vi "Zernike_to_Motion.vi"(0 "HasoSlopes in":refnum<class "HasoSlopes.lvclass">, 1 "CorrectionDataManager (const)":refnum<class "CorrectionDataManager.lvclass">, 2 "Pupil (const)":refnum<class "Pupil.lvclass">, 3 "WavefrontCorrector in":refnum<class "WavefrontCorrector.lvclass">, 4 "ComputePhaseSet":refnum<class "ComputePhaseSet.lvclass">, 5 "error in (no error)":errorcluster, 6 "radius":sgl, 7 "ModalCoef (const)":refnum<class "ModalCoef.lvclass">, 8 "center":T1, 9 "Prefs in":T2={"Number of kept modes"=32, "Tilt filtering"=FALSE}, 10 "ZernikeArray":dbl[](array[numeric])) -> (12 "CorrectionDataManager out":refnum<class "CorrectionDataManager.lvclass">, 13 "Delta commands 2":sgl[](graph), 14 "HasoSlopes out":refnum<class "HasoSlopes.lvclass">, 15 "Pupil (dup)":refnum<class "Pupil.lvclass">, 16 "WavefrontCorrector out":refnum<class "WavefrontCorrector.lvclass">, 17 "ComputePhaseSet (dup)":refnum<class "ComputePhaseSet.lvclass">, 18 "ModalCoef.lvclass (dup)":refnum<class "ModalCoef.lvclass">, 19 "error out":errorcluster)   [LabVIEW 2020, in "ILAO_BeamShaper.lvclass"]
uses:
  ILAO_BeamShaper.lvclass
  HASO4_3/WaveKit/Controls/InteractionMatrixToCommandMatrixParameters.ctl
  HASO4_3/WaveKit/Classes/Pupil/Pupil.lvclass
  HASO4_3/WaveKit/Classes/WavefrontCorrector/WavefrontCorrector.lvclass
  HASO4_3/WaveKit/Classes/ModalCoef/ModalCoef.lvclass
  HASO4_3/WaveKit/Classes/ComputePhaseSet/ComputePhaseSet.lvclass
  HASO4_3/WaveKit/Classes/CorrectionDataManager/CorrectionDataManager.lvclass
  HASO4_3/WaveKit/Classes/HasoSlopes/HasoSlopes.lvclass
  HASO4_3/WaveKit/Controls/Point2Df.ctl
  HASO4_3/WaveKit/Controls/ZernikeModalPrefs.ctl
  HASO4_3/WaveKit/Controls/ZernikeProjectionPupilSetup.ctl
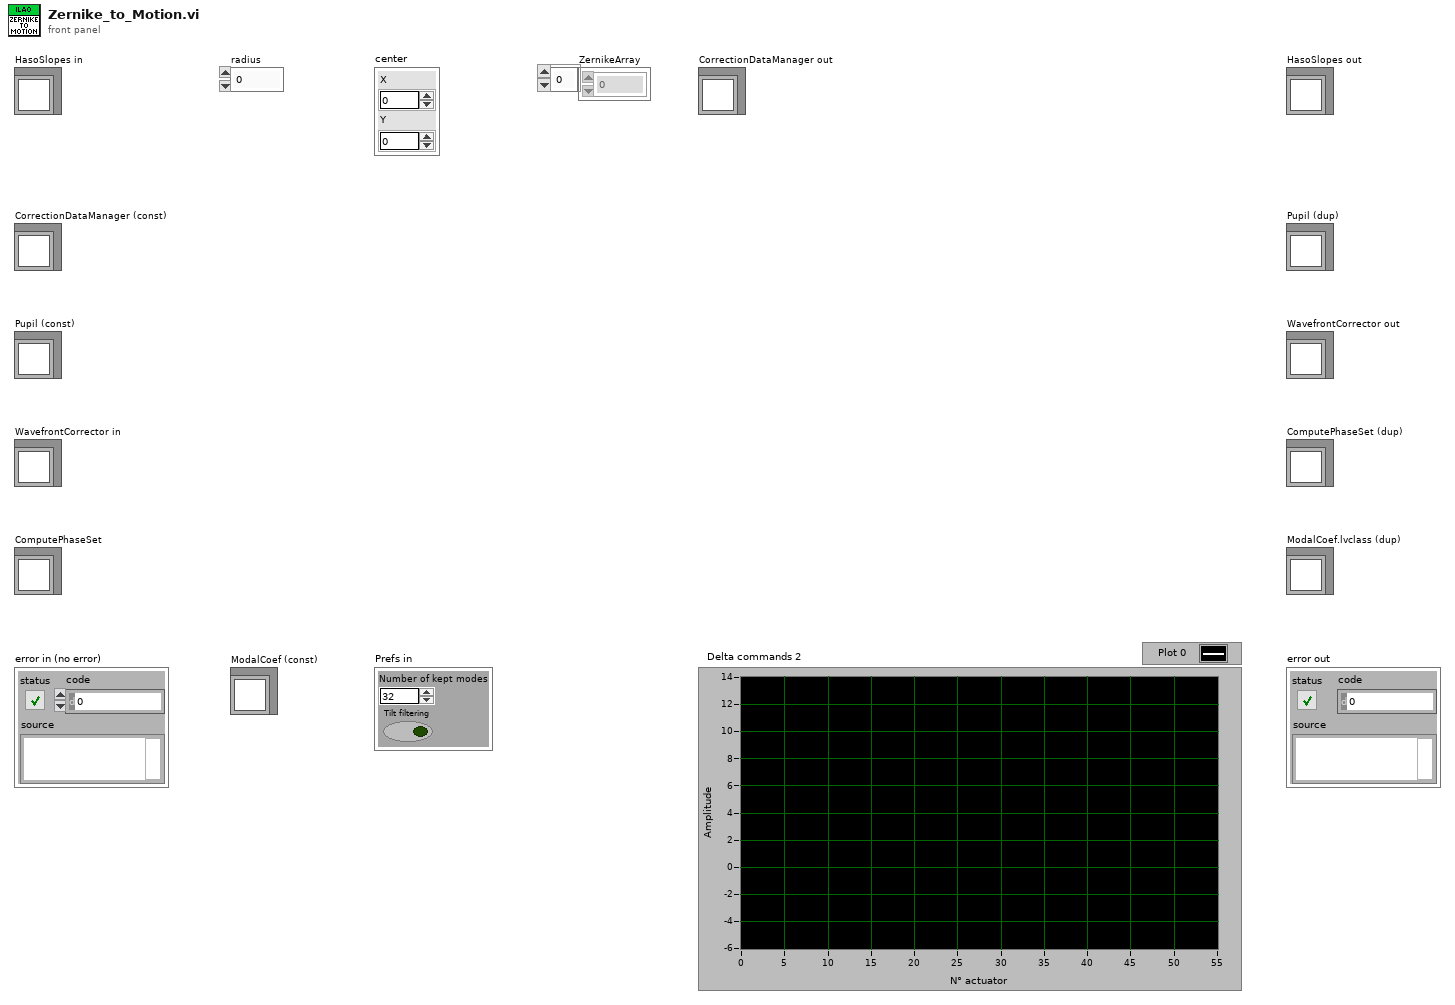
[diagram p1: front panel]
types:
  T1 = typedef "Point2Df.ctl" = cluster{"X":sgl, "Y":sgl}
  T2 = typedef "InteractionMatrixToCommandMatrixParameters.ctl" = cluster{"Number of kept modes":i32, "Tilt filtering":bool}
  T3 = typedef "ZernikeModalPrefs.ctl" = cluster{"Number of coefficients":u32, "Filtered coefficients":u32[], "RMS Zernike normalization":bool, "CircularProjectionPupilDimensions":T4}
  T4 = typedef "ZernikeProjectionPupilSetup.ctl" = cluster{"Pupil center_sspp":T1, "Pupil radius_sspp":sgl}
  T5 = typedef "Wavefront Corrector Position.ctl" = sgl[]
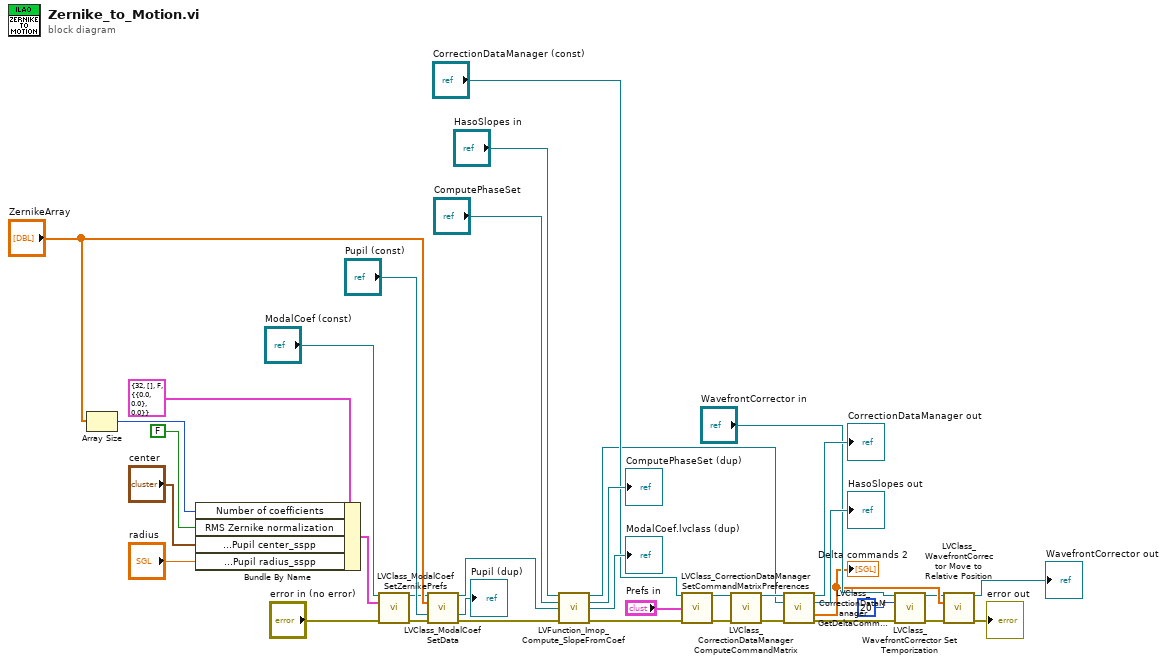
[diagram p0: block diagram]
diagram:
  n1 = Array Size(array="ZernikeArray") -> (size(s)=w1:i32)
  n2 = Bundle By Name(cluster=T3 {"Number of coefficients"=32, "Filtered coefficients"=[], "RMS Zernike normalization"=FALSE, "CircularProjectionPupilDimensions"={"Pupil center_sspp"={"X"=0.0, "Y"=0.0}, "Pupil radius_sspp"=0.0}} ("ZernikeModalPrefs 2"), "Number of coefficients"=w1, "RMS Zernike normalization"=FALSE, "CircularProjectionPupilDimensions.Pupil center_sspp"="center", "CircularProjectionPupilDimensions.Pupil radius_sspp"="radius") -> (w3:T3)
  n3 = call "LVClass_ModalCoef SetZernikePrefs.vi"("ModalCoef in"="ModalCoef (const)", "ZernikeModalPrefs"=w3, "error in (no error)"="error in (no error)") -> ("ModalCoef out"=w4:refnum<class "ModalCoef.lvclass">, "error out"=w32:errorcluster)  [unwired: 11 in]
  n4 = call "LVClass_ModalCoef SetData.vi"("ModalCoef in"=w4, "coef"="ZernikeArray", "Pupil.lvclass"="Pupil (const)", "error in (no error)"=w32) -> ("ModalCoef out"=w5:refnum<class "ModalCoef.lvclass">, "Pupil (dup)"=→"Pupil (dup)":refnum<class "Pupil.lvclass">, "error out"=w33:errorcluster)  [unwired: 8 in, 1 out]
  n5 = call "LVFunction_Imop_Compute_SlopeFromCoef.vi"("HasoSlopes.lvclass"="HasoSlopes in", "ComputePhaseSet"="ComputePhaseSet", "ModalCoef.lvclass"=w5, "error IO"=w33) -> ("HasoSlopes.lvclass"=w9:refnum<class "HasoSlopes.lvclass">, "ComputePhaseSet (dup)"=→"ComputePhaseSet (dup)":refnum<class "ComputePhaseSet.lvclass">, "ModalCoef.lvclass (dup)"=→"ModalCoef.lvclass (dup)":refnum<class "ModalCoef.lvclass">, "error IO out"=w34:errorcluster)  [unwired: 8 in]
  n6 = call "LVClass_CorrectionDataManager SetCommandMatrixPreferences.vi"("CorrectionDataManager in"="CorrectionDataManager (const)", "Prefs"="Prefs in", "error in (no error)"=w34) -> ("CorrectionDataManager out"=w10:refnum<class "CorrectionDataManager.lvclass">, "error out"=w7:errorcluster)  [unwired: 11 in]
  n7 = call "LVClass_CorrectionDataManager ComputeCommandMatrix.vi"("CorrectionDataManager in"=w10, "error in (no error)"=w7) -> ("CorrectionDataManager out"=w11:refnum<class "CorrectionDataManager.lvclass">, "error out"=w6:errorcluster)  [unwired: 12 in]
  n8 = call "LVClass_CorrectionDataManager GetDeltaCommandsFromDeltaSlopes.vi"("CorrectionDataManager in"=w11, "Delta Slopes IN"=w9, "error in (no error)"=w6) -> ("CorrectionDataManager out"=→"CorrectionDataManager out":refnum<class "CorrectionDataManager.lvclass">, "Delta Slope OUT"=→"HasoSlopes out":refnum<class "HasoSlopes.lvclass">, "DeltaPosition"=w13:T5, "error out"=w36:errorcluster)  [unwired: 9 in]
  "Delta commands 2" <- w13
  n9 = call "LVClass_WavefrontCorrector Set Temporization.vi"("WavefrontCorrector in"="WavefrontCorrector in", "Sleep after command apply (ms)"=20, "error in (no error)"=w36) -> ("WavefrontCorrector out"=w12:refnum<class "WavefrontCorrector.lvclass">, "error out"=w37:errorcluster)  [unwired: 11 in]
  n10 = call "LVClass_WavefrontCorrector Move to Relative Position.vi"("WavefrontCorrector in"=w12, "Wavefront Relative Position"=w13, "error in (no error)"=w37) -> ("WavefrontCorrector out"=→"WavefrontCorrector out":refnum<class "WavefrontCorrector.lvclass">, "error out"=→"error out":errorcluster)  [unwired: 11 in]
